vi "Robot Global Data V.5.0.vi"() -> ()   [LabVIEW 2016]
doc: "This global VI can contain as many global variables as you need. Place a control on the panel, give it a good name. To read or write to it from a VI, drag the icon to the diagram of that VI. You can also drag from the project. Click on the node to change which global you access. You shouldn't have multiple locations writing to a global or it will cause a race-condition."
uses:
  <vilib>/Rock Robotics/WPI/Camera/WPI_CameraImageSize.ctl
  <vilib>/Rock Robotics/WPI/DriverStation/WPI_DriverStationRobotMode2.ctl
panel:
  in  "False = Mid Cam & True = Side Cam":bool
  out "Auto Turning State":string
  in  "Servo":dbl
  in  "False = Reg. Expo. & True = Low Expo.":bool
  in  "Teleop Encoder Reset Iteration Counter":dbl
  out "Drive Trigger Speed Change":dbl
  in  "Gear Holder Open":bool
  out "Gear Gobbler Y":dbl
  in  "Ball Dumper Open":bool
  out "Compressor On?":bool
  out "Compressor Enabled?":bool
  in  "Gear State":string
  in  "Climbing Nudge":bool
  in  "Climbing Talon Current":dbl
  in  "Inside Switch":bool
  in  "Frame Switch":bool
  in  "Constant Climbing":bool
  out "Gyro":dbl
  out "Right Encoder Start":dbl
  out "Left Encoder Start":dbl
  in  "Right Speed Fix":dbl
  in  "Left Speed Fix":dbl
  in  "Veering Iteration Counter":dbl
  out "Right Encoder":dbl
  out "Left Encoder":dbl
  out "Right Joystick Y":dbl
  out "Left Joystick X":dbl
  out "Left Joystick Y":dbl
  out "Right Joystick X":dbl
  in  "Tank = False & Arcade = True":bool
  in  "Robot Mode":T1
  out "ms to process":u32
  out "Vision Results":T2 {"Score" format="%#_3g"; "Pixels"."Rectangle"."Numeric 5" format="%#_3g"; "Pixels"."Rectangle"."Numeric 3" format="%#_3g"; "Pixels"."Rectangle"."Numeric 2" format="%#_3g"; "Pixels"."Rectangle"."Numeric" format="%#_3g"; "Normalized"."Rectangle"."Numeric 5" format="%#_2g"; "Normalized"."Rectangle"."Numeric 3" format="%#_2g"; "Normalized"."Rectangle"."Numeric 2" format="%#_2g"; "Normalized"."Rectangle"."Numeric" format="%#_2g"; "Normalized"."Center"."?" format="%#_3g"; "Normalized"."Center"."?" format="%#_3g"; "Distance (ft)" format="%#_3g"}
  in  "image size":T3=enum."320x240"
  in  "Enable Vision":bool
  # "Encoder values in feet"
  # "Encoder  values when begin runs"
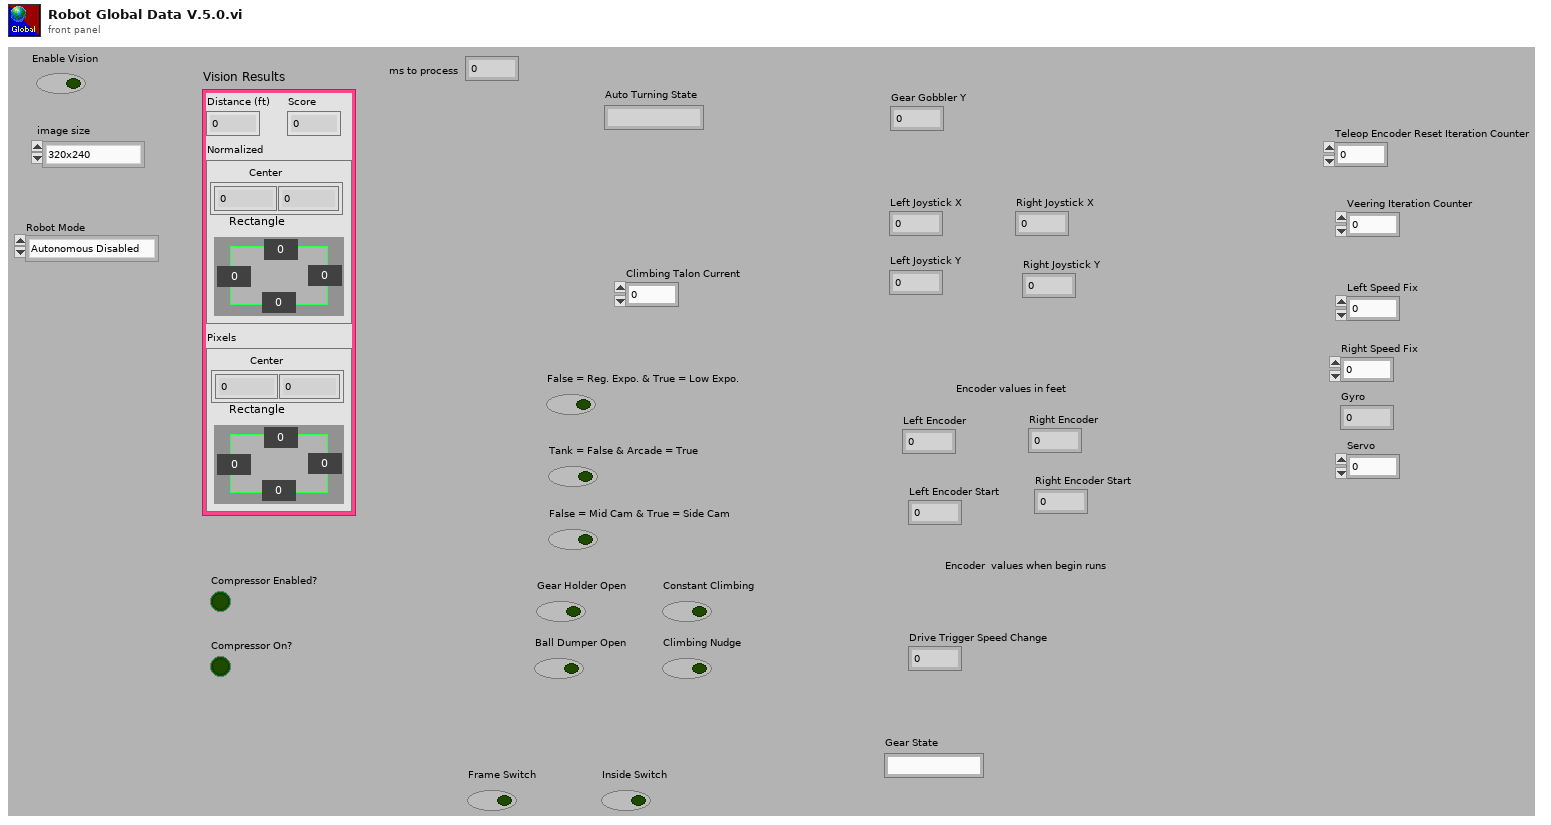
[diagram p1: front panel]
types:
  T1 = typedef "WPI_DriverStationRobotMode2.ctl" = enum16{"Autonomous Disabled", "Autonomous Enabled", "Teleop Disabled", "Teleop Enabled", "Disconnected", "Finish", "Test Disabled", "Test Enabled", "Emergency Stopped"}
  T2 = cluster{"Distance (ft)":dbl, "Score":dbl, "Normalized":cluster{"Center":cluster{dbl, dbl}, "Rectangle":cluster{"Numeric":dbl, "Numeric 2":dbl, "Numeric 3":dbl, "Numeric 5":dbl}}, "Pixels":cluster{"Center":cluster{dbl, dbl}, "Rectangle":cluster{"Numeric":dbl, "Numeric 2":dbl, "Numeric 3":dbl, "Numeric 5":dbl}}}
  T3 = typedef "WPI_CameraImageSize.ctl" = enum16{"640x480", "320x240", "160x120", "Custom"}
diagram:
